vi "read_acq_mode.vi"(8 "error in (no error)":errorcluster, 11 "hydraharp in":refnum<class "hydraharp.lvclass">) -> (0 "error out":errorcluster, 2 "Mode":T1 items=["T2"=2, "T3"=3], 3 "hydraharp out":refnum<class "hydraharp.lvclass">)   [LabVIEW 2015, in "hydraharp.lvclass"]
uses:
  hydraharp.lvclass
  hydraharp_panel/hpanel_acq_modes.ctl
  hydraharp.lvclass/hydraharp.ctl
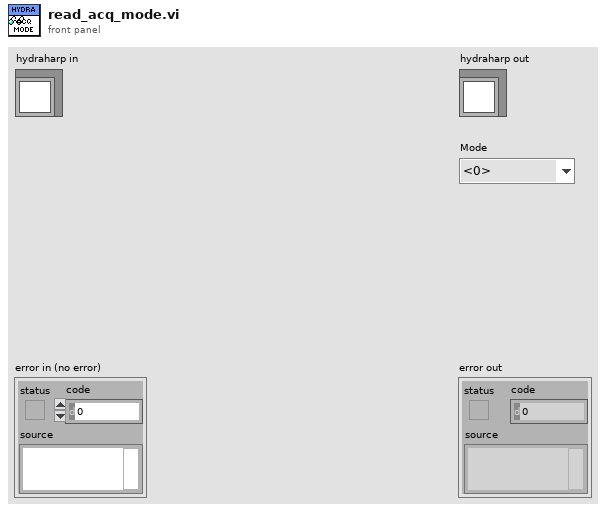
[diagram p1: front panel]
types:
  T1 = typedef "hpanel_acq_modes.ctl" = u16
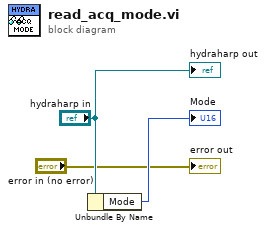
[diagram p0: block diagram]
diagram:
  n1 = Unbundle By Name("hydraharp in") -> ("Mode"=→"Mode":T1)
  "error out" <- "error in (no error)"
  "hydraharp out" <- "hydraharp in"
